vi "LabviewPython.vi"() -> ()   [LabVIEW 2022 SP3]
panel:
  out "Value":T1
  out "Initial message":string
  out "Current Data":dbl
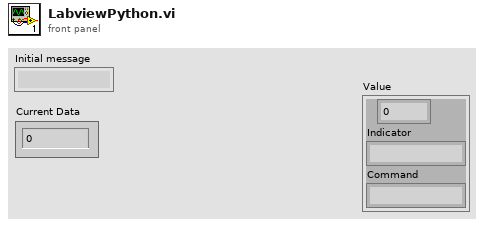
[diagram p1: front panel]
types:
  T1 = cluster{dbl, "Indicator":string, "Command":string}
  T2 = enum16{"SCAN", "TDC", "CAM", "POW", "LOG", "ANLYS", "VOLT", "MOTOR", "DELAY", "LASER"}
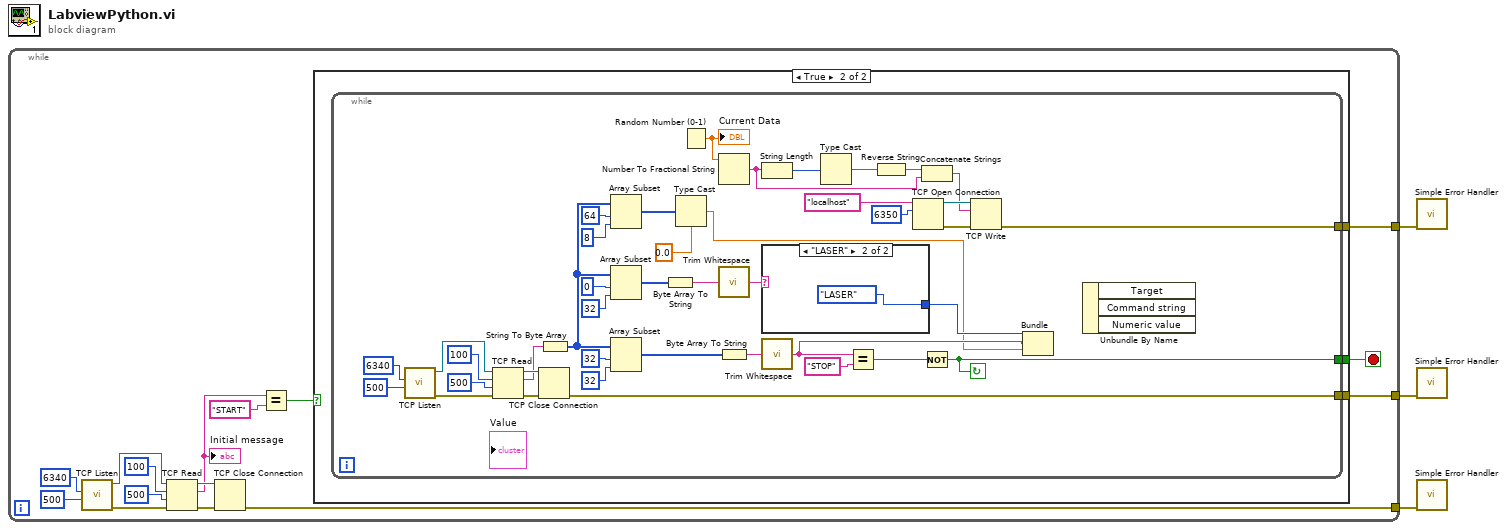
[diagram p0: block diagram]
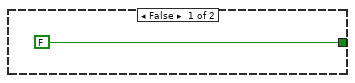
[diagram p2: hidden frame]
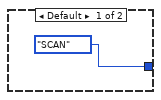
[diagram p3: hidden frame]
diagram:
  n1 = while {
    tunnel: [w6] -> w3
    tunnel: [w5] -> w2
    tunnel: [w4] -> w1
    stop <- w7 stop-if-true
    n2 = call <vilib>:"TCP Listen.vi"("timeout ms (wait forever: -1)"=500, "port"=u16 6340 ("remote port or service name")) -> ("error out"=w15:errorcluster, "connection ID"=w16:refnum<k5>)  [unwired: 5 in, 3 out]
    n3 = TCP Read(connection ID=w16, bytes to read=100, error in (no error)=w15, 9:500 ("timeout ms (25000)")) -> (connection ID out=w13:refnum<k5>, data out=w10:string, error out=w12:errorcluster)  [unwired: 1 in]
    "Initial message" <- w10
    n4 = TCP Close Connection(connection ID=w13, error in (no error)=w12) -> (error out=w4:errorcluster)  [unwired: 1 in, 1 out]
    n5 = Equal?(x=w10, y="START") -> (x = y?=w8:bool)
    n6 = case shown="True" w8 {
      tunnel: [FALSE w22] -> w7
      tunnel: [_ w21] -> w6
      tunnel: [_ w20] -> w5
      frame False {
      }
      frame True {
        n7 = while {
          tunnel: [w61] -> w21
          tunnel: [w50] -> w20
          tunnel: [w41] -> w22
          stop <- w41 continue-if-true
          n8 = call <vilib>:"TCP Listen.vi"("timeout ms (wait forever: -1)"=500, "port"=u16 6340 ("remote port or service name")) -> ("error out"=w59:errorcluster, "connection ID"=w60:refnum<k5>)  [unwired: 5 in, 3 out]
          n9 = TCP Read(connection ID=w60, bytes to read=100, error in (no error)=w59, 9:500 ("timeout ms (25000)")) -> (connection ID out=w57:refnum<k5>, data out=w40:string, error out=w56:errorcluster)  [unwired: 1 in]
          n10 = TCP Close Connection(connection ID=w57, error in (no error)=w56) -> (error out=w61:errorcluster)  [unwired: 1 in, 1 out]
          n11 = String To Byte Array(string=w40) -> (unsigned byte array=w33:u8[])
          n12 = Array Subset(array=w33, index=64, length=8) -> (w30:u8[])
          n13 = Array Subset(array=w33, index=0, length=32) -> (w32:u8[])
          n14 = Array Subset(array=w33, index=32, length=32) -> (w31:u8[])
          n15 = Byte Array To String(unsigned byte array=w32) -> (string=w28:string)
          n16 = Type Cast(type=0.0, x=w30) -> (*(type *) &x=w24:dbl)
          n17 = Random Number (0-1)() -> (number: 0 to 1=w44:dbl)
          "Current Data" <- w44
          n18 = Number To Fractional String(number=w44) -> (F-format string=w49:string)  [unwired: 3 in]
          n19 = call <vilib>:"Trim Whitespace.vi"("string"=w28) -> ("trimmed string"=w27:string)  [unwired: 1 in]
          n20 = Byte Array To String(unsigned byte array=w31) -> (string=w29:string)
          n21 = String Length(string=w49) -> (length=w46:i32)
          n22 = case shown="\"LASER\"" w27 {
            tunnel: [T2."SCAN" ("Target") T2."LASER" ("Target")] -> w26
            frame Default {
            }
            frame "LASER" {
            }
          }
          n23 = call <vilib>:"Trim Whitespace.vi"("string"=w29) -> ("trimmed string"=w25:string)  [unwired: 1 in]
          n24 = Type Cast(x=w46) -> (*(type *) &x=w47:string)  [unwired: 1 in]
          n25 = Equal?(x=w25, y="STOP") -> (x = y?=w42:bool)
          n26 = Reverse String(1:w47) -> (0:w48:string)
          n27 = TCP Open Connection(address="localhost", remote port or service name=u16 6350) -> (connection ID=w54:refnum<k5>, error out=w53:errorcluster)  [unwired: 3 in]
          n28 = Concatenate Strings(w48, w49) -> (w45:string)
          n29 = Not(x=w42) -> (.not. x?=w41:bool)
          n30 = TCP Write(connection ID=w54, data in=w45, error in (no error)=w53) -> (error out=w50:errorcluster)  [unwired: 1 in, 2 out]
          n31 = Bundle("Target"=w26, "trimmed string"=w25, w24) -> ()  [unwired: 1 in, 1 out]
          n32 = Unbundle By Name() -> ()  [unwired: 1 in, 3 out]
        }
      }
    }
  }
  n33 = call <vilib>:"Simple Error Handler.vi"("error in (no error)"=w2) -> ()  [unwired: 4 in, 5 out]
  n34 = call <vilib>:"Simple Error Handler.vi"("error in (no error)"=w3) -> ()  [unwired: 4 in, 5 out]
  n35 = call <vilib>:"Simple Error Handler.vi"("error in (no error)"=w1) -> ()  [unwired: 4 in, 5 out]
